vi "Error.vi"(8 "error in (no error)":errorcluster, 10 "error":errorcluster, 11 "Sample Error Manager in":refnum<class "Sample Error Manager.lvclass">) -> (0 "error out":errorcluster, 3 "Sample Error Manager out":refnum<class "Sample Error Manager.lvclass">)   [LabVIEW 2024, in "Sample Error Manager.lvlib" / "Sample Error Manager.lvclass"]
uses:
  Sample Error Manager.lvclass
  Sample Error Manager.lvclass/Sample Error Manager.ctl
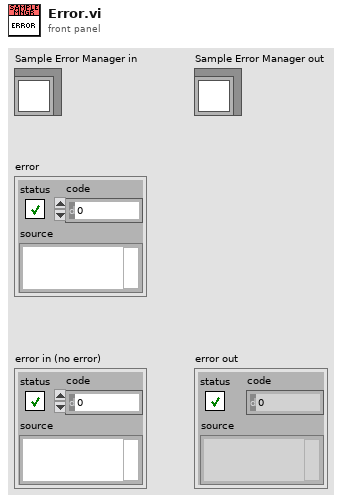
[diagram p1: front panel]
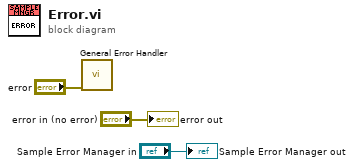
[diagram p0: block diagram]
diagram:
  n1 = call <vilib>:"General Error Handler.vi"("error in (no error)"="error") -> ()  [unwired: 10 in, 5 out]
  "error out" <- "error in (no error)"
  "Sample Error Manager out" <- "Sample Error Manager in"
